vi "Entering_State.vi"(8 "error in":errorcluster, 10 "State_Info":T1, 11 "Parameters to process":T6) -> (0 "error out":errorcluster, 1 "Results from processing":T5, 2 "State_Info_Out":T1)   [LabVIEW 2017, in "ExampleSequencer runtime.lvclass"]
uses:
  ExampleSequencer runtime.lvclass
  parameter user data.ctl
  result user data.ctl
  State.ctl
  Utilities/StateMachine.ctl
  <vilib>/NI/STM/TCP/TCP Connection Info.ctl
  <vilib>/NI/STM/SubVIs/MetaDataElement.ctl
  Utilities/WordManipulationLibrary.lvlib
  <vilib>/NI/STM/NI STM.lvlib
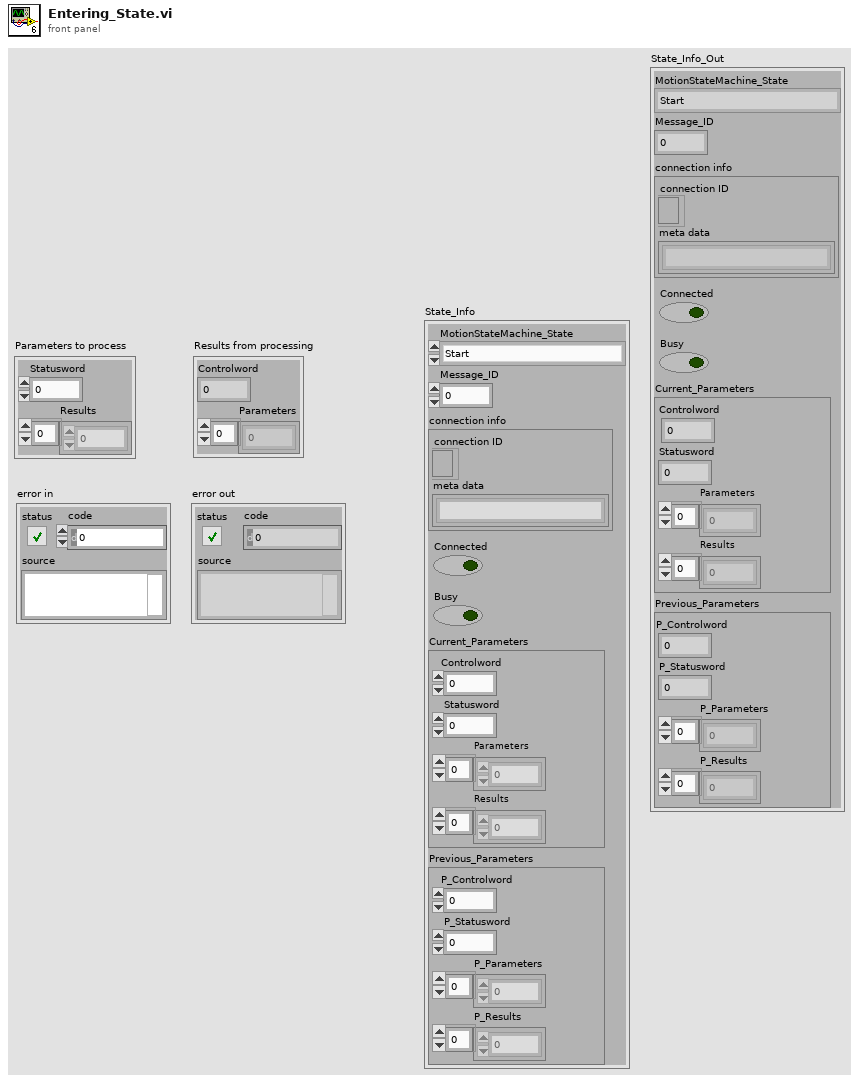
[diagram p1: front panel]
types:
  T1 = typedef "State.ctl" = cluster{"MotionStateMachine_State":T2, "Message_ID":u32, "connection info":T3, "Connected":bool, "Busy":bool, "Current_Parameters":cluster{"Controlword":u16, "Statusword":u16, "Parameters":dbl[], "Results":dbl[]}, "Previous_Parameters":cluster{"P_Controlword":u16, "P_Statusword":u16, "P_Parameters":dbl[], "P_Results":dbl[]}}
  T2 = typedef "WordManipulationLibrary.lvlib/StateMachine.ctl" = enum16{"Start", "Not Ready to Switch On", "Switch On Disabled", "Ready to Switch On", "Switched On", "Operation enable", "Quick Stop Active", "Fault Reaction Active", "Fault"}
  T3 = typedef "NI STM.lvlib/TCP Connection Info.ctl" = cluster{"connection ID":refnum<k5>, "meta data":T4[]}
  T4 = typedef "NI STM.lvlib/MetaDataElement.ctl" = string
  T5 = typedef "ExampleSequencer runtime.lvclass/result user data.ctl" = cluster{"Controlword":u16, "Parameters":dbl[]}
  T6 = typedef "ExampleSequencer runtime.lvclass/parameter user data.ctl" = cluster{"Statusword":u16, "Results":dbl[]}
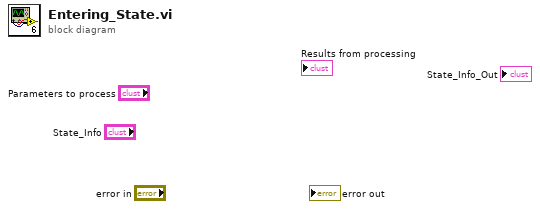
[diagram p0: block diagram]
diagram:
